vi "convert color string summary.vi"(1 "primary":u32(colorbox)) -> (0 "String":string)   [LabVIEW 2021, in "TSC Material Theme.lvlib" / "Material-Scheme.lvclass"]
doc: "Define the tip strip info for the Scheme -> adds the hex and RGB info to the string\n\n<b>Code Developed By:</b> +\nDaniel Coons +\nTechnology Service Corporation +\nwww.tsc.com/atcs"
uses:
  Material-Scheme.lvclass
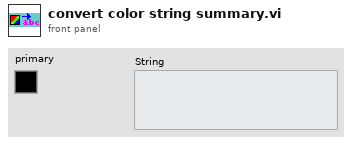
[diagram p1: front panel]
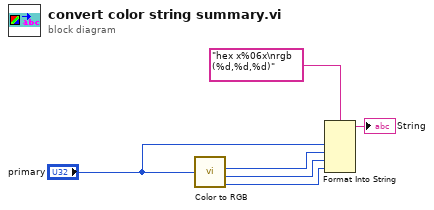
[diagram p0: block diagram]
diagram:
  n1 = call <vilib>:"Color to RGB.vi"("Color"="primary") -> ("R"=w2:u8, "G"=w3:u8, "B"=w4:u8)  [unwired: 1 out]
  n2 = Format Into String(format string="hex x%06x\nrgb (%d,%d,%d)", "primary", w2, w3, w4) -> (resulting string=→"String":string)  [unwired: 2 in, 1 out]
